vi "1_Analog_Meter_Reader(Training).vi"() -> ()   [LabVIEW 2020]
doc: "This example demonstrating the usage of Deep Learning toolkit for solving geometrical objects recognition problem based on Multilayer perceptron (MLP) and Convolutional Neural Network (CNN)."
uses:
  <vilib>/Ngene/DeepLTK/Toolkit/NN_Train/Controls/NN_LR_Policy_Cfg.ctl
  <vilib>/Ngene/DeepLTK/Toolkit/NN_Train/Controls/NN_LR_Policy_Type.ctl
  <vilib>/Ngene/DeepLTK/Toolkit/NN_Train/Controls/NN_Train_Params.ctl
  <vilib>/Ngene/DeepLTK/Toolkit/NN_Train/Controls/NN_Train_Optimizer.ctl
  <vilib>/Ngene/DeepLTK/Toolkit/NN_Train/Controls/NN_Train_Data_Sampling.ctl
  Controls/Regression_Report.ctl
  <vilib>/Ngene/DeepLTK/Toolkit/NN_Layers/Layers/FC/Controls/NN_Layer_Config(FC).ctl
  <vilib>/Ngene/DeepLTK/Toolkit/NN_Layers/Layers/BatchNorm/Controls/NN_BN_Params.ctl
  <vilib>/Ngene/DeepLTK/Toolkit/NN_Activations/Controls/NN_Activation_Type.ctl
  <vilib>/Ngene/DeepLTK/Toolkit/NN_Layers/Controls/NN_Layer_Init_Params.ctl
  <vilib>/Ngene/DeepLTK/Toolkit/NN_Layers/Controls/NN_Layer_Weight_Init_Type.ctl
  <vilib>/Ngene/DeepLTK/Toolkit/NN_Layers/Layers/Input/Controls/NN_Layer_Config(Input3D).ctl
  <vilib>/Ngene/DeepLTK/Toolkit/NN_Data/Controls/NN_Dims(C,H,W).ctl
  <vilib>/Ngene/DeepLTK/Toolkit/NN_Network/Controls/NN_Save_Before_Destroy_Options.ctl
  <vilib>/Ngene/DeepLTK/Toolkit/NN_Layers/Layers/Conv2D/Controls/NN_Layer_Config(Conv2D).ctl
  <vilib>/Ngene/DeepLTK/Toolkit/NN_Layers/Layers/Conv2D/Controls/NN_Layer_Params(Conv2D).ctl
  <vilib>/Ngene/DeepLTK/Toolkit/NN_Layers/Layers/Conv2D/Controls/NN_Conv2D_Padding_Type.ctl
  <vilib>/Ngene/DeepLTK/Toolkit/NN_Layers/Layers/DropOut3D/Controls/NN_Layer_Config(DropOut3D).ctl
  <vilib>/Ngene/DeepLTK/Toolkit/NN_Layers/Layers/Input/NN_Layer_Create(Input3D).vi
  <vilib>/Ngene/DeepLTK/Toolkit/NN_Layers/Layers/Conv2D/NN_Layer_Create(Conv2D).vi
  <vilib>/Ngene/DeepLTK/Toolkit/NN_Layers/Layers/DropOut3D/NN_Layer_Create(DropOut3D).vi
  <vilib>/Ngene/DeepLTK/Toolkit/NN_Layers/Layers/FC/NN_Layer_Create(FC).vi
  <vilib>/Ngene/DeepLTK/Toolkit/NN_Train/Loss_Functions/NN_Set_Loss(MSE).vi
  <vilib>/ptbypt/Filters.llb/FIR Filter PtByPt.vi
  <vilib>/Ngene/DeepLTK/Toolkit/NN_Network/subVIs/NN_Predict/NN_Predict(In3D_Out1D).vi
  <vilib>/Ngene/DeepLTK/Toolkit/NN_Train/Eval_Loss/NN_Eval_Test_Error_Loss/NN_Eval(In3D_Out1D).vi
  <vilib>/Ngene/DeepLTK/Toolkit/NN_Data/subVIs/Dataset_Destroy/NN_Datasets_All_Destroy(In3D_Out1D).vi
  <vilib>/Ngene/DeepLTK/Toolkit/Deep_Learning_Toolkit_by_Ngene.lvlib
panel:
  in  "NN Device":enum16{"CPU", "GPU"}(ring)=enum."GPU"
  out "Train Speed (img/s)":dbl=2338.672694098055 format="%#_3p"
  out "Train Speed (sec/batch)":dbl=0.10946379997767508 format="%#_3p"
  out "Elapsed Time":dbl=32.9020060999901 format="%<%H:%M:%S>t"
  out "Test.Dataset_Size":i32=201
  out "Train.Dataset_Size":i32=1000
  out "Loss Values":cluster{"Train_Loss":dbl, "Test_Loss":dbl}={"Train_Loss"=7.778966903686523, "Test_Loss"=0.4036712646484375} {"Test_Loss" format="%#_4g"}
  out "Session Data":T1={"Epochs"=104.19200134277344, "Tot_Iter"=407.0, "LR"=9.5367431640625e-06, "LR_iter"=408.0} {"LR" format="%#_3g"}
  out "Loss Charts":cluster{"Filtered x":sgl, "Test_Loss":sgl}(graph)={"Filtered x"=7.778967, "Test_Loss"=0.40367126}
  in  "Image Folder(Test)":path=path "D:/working/Analog_Meter/Test/Images"
  in  "Labels (Test)":path=path "D:/working/Analog_Meter/Test/Labels.csv"
  in  "Stop":bool
  out "Regression Metrics":T2={"Graphs"=[{"Best Linear Fit"=array[201 elements], "Array 3"=[2.517011, 2.0096045, 2.4545722, 2.2636914, 2.2936764, 4.560302, 5.5319304, 6.4831433, 6.3087363, 7.618647, 8.221905, 9.112002, 9.980037, 9.071789, 9.958405, 10.536366, 11.692846, 12.491657, 13.6740055, 14.302982, 14.830361, 15.396115, 15.868366, 16.362938, 16.752916, 17.515846, 18.169603, 18.99068, 19.849512, 20.732693, 21.52332, 22.002708, 22.214579, 23.227516, 24.120646, 25.386911, 25.468521, 26.268867, 27.2104, 28.526808, 28.953384, 29.351616, 29.946152, 30.505703, 31.088083, 31.950428, 32.824123, 33.49473, 34.381035, 35.134453, 35.577026, 36.282093, 36.62258, 37.27366, 37.827774, 39.678932, 40.030205, 40.623016, 41.345863, 41.777946, 42.25227, 42.78178, 43.344627, 44.43666, 45.447147, 46.357304, 47.180454, 47.77743, 48.22017, 48.731907, 49.320972, 50.022675, 50.477943, 51.13582, 51.981068, 52.795086, 53.414444, 54.063515, 54.653965, 56.161224, 56.6563, 57.51746, 58.014706, 58.689663, 59.56889, 60.116806, 60.655125, 61.062958, 61.754738, 62.627365, 63.322636, 63.751377, 64.42173, 65.163635, 65.93629, 67.140495, 67.96894, 68.54193, 69.32477, 69.879906, 70.43094, 71.16161, 71.60928, 72.36131, 72.99475, 73.651764, 74.624405, 75.3703, 76.09268, 76.79159, 77.39567, 78.15343, 78.86843, 79.65233, 80.15797, 80.81467, 81.317024, 82.1362, 82.814064, 83.34939, 84.02449, 84.577354, 86.16109, 86.68068, 87.33571, 88.01903, 88.70086, 89.229324, 89.99918, 90.731285, 91.37161, 92.006744, 92.70506, 93.25279, 94.06685, 94.801796, 95.546906, 96.167404, 97.10623, 97.73104, 98.33137, 98.990654, 99.54073, 100.25781, 100.895294, 101.526665, 102.33004, 102.97929, 103.77419, 104.16804, 104.88838, 106.019455, 106.816345, 107.406876, 108.19176, 109.02587, 109.658844, 110.24592, 110.704124, 111.26262, 111.76719, 112.43235, 113.87547, 114.76889, 115.557724, 115.86315, 116.95176, 117.768394, 118.702324, 118.6948, 119.12609, 119.788155, 120.696465, 121.51759, 122.282455, 122.96412, 123.52434, 124.11557, 124.71953, 125.29246, 125.93008, 126.66733, 127.38417, 128.6919, 129.43976, 130.39424, 131.04564, 131.64711, 131.56487, 132.2587, 133.19635, 133.81221, 134.28249, 134.72006, 135.67499, 136.66454, 138.42493, 138.63422, 138.48953, 138.73322, 137.90044]}, {"Best Linear Fit"=array[201 elements], "Array 3"=[2.517011, 2.0096045, 2.4545722, 2.2636914, 2.2936764, 4.560302, 5.5319304, 6.4831433, 6.3087363, 7.618647, 8.221905, 9.112002, 9.980037, 9.071789, 9.958405, 10.536366, 11.692846, 12.491657, 13.6740055, 14.302982, 14.830361, 15.396115, 15.868366, 16.362938, 16.752916, 17.515846, 18.169603, 18.99068, 19.849512, 20.732693, 21.52332, 22.002708, 22.214579, 23.227516, 24.120646, 25.386911, 25.468521, 26.268867, 27.2104, 28.526808, 28.953384, 29.351616, 29.946152, 30.505703, 31.088083, 31.950428, 32.824123, 33.49473, 34.381035, 35.134453, 35.577026, 36.282093, 36.62258, 37.27366, 37.827774, 39.678932, 40.030205, 40.623016, 41.345863, 41.777946, 42.25227, 42.78178, 43.344627, 44.43666, 45.447147, 46.357304, 47.180454, 47.77743, 48.22017, 48.731907, 49.320972, 50.022675, 50.477943, 51.13582, 51.981068, 52.795086, 53.414444, 54.063515, 54.653965, 56.161224, 56.6563, 57.51746, 58.014706, 58.689663, 59.56889, 60.116806, 60.655125, 61.062958, 61.754738, 62.627365, 63.322636, 63.751377, 64.42173, 65.163635, 65.93629, 67.140495, 67.96894, 68.54193, 69.32477, 69.879906, 70.43094, 71.16161, 71.60928, 72.36131, 72.99475, 73.651764, 74.624405, 75.3703, 76.09268, 76.79159, 77.39567, 78.15343, 78.86843, 79.65233, 80.15797, 80.81467, 81.317024, 82.1362, 82.814064, 83.34939, 84.02449, 84.577354, 86.16109, 86.68068, 87.33571, 88.01903, 88.70086, 89.229324, 89.99918, 90.731285, 91.37161, 92.006744, 92.70506, 93.25279, 94.06685, 94.801796, 95.546906, 96.167404, 97.10623, 97.73104, 98.33137, 98.990654, 99.54073, 100.25781, 100.895294, 101.526665, 102.33004, 102.97929, 103.77419, 104.16804, 104.88838, 106.019455, 106.816345, 107.406876, 108.19176, 109.02587, 109.658844, 110.24592, 110.704124, 111.26262, 111.76719, 112.43235, 113.87547, 114.76889, 115.557724, 115.86315, 116.95176, 117.768394, 118.702324, 118.6948, 119.12609, 119.788155, 120.696465, 121.51759, 122.282455, 122.96412, 123.52434, 124.11557, 124.71953, 125.29246, 125.93008, 126.66733, 127.38417, 128.6919, 129.43976, 130.39424, 131.04564, 131.64711, 131.56487, 132.2587, 133.19635, 133.81221, 134.28249, 134.72006, 135.67499, 136.66454, 138.42493, 138.63422, 138.48953, 138.73322, 137.90044]}, {"Best Linear Fit"=[0.0, 140.0], "Array 3"=[0.0, 140.0]}], "y=k*x+b"="y = 0.996*x + 0.683", "R"=0.9999493, "R^2"=0.99989855, "MAE"=0.46021813, "MSE"=0.3585698} {"R" format="%#_7g"}
  in  "Evaluate Model":bool
  in  "LR Update Policy":T3={"Policy_Type"=enum."Step", "LR0"=10.0, "k"=5.0, "WarmUp_Policy"=enum."Ramp", "WarmUp_Iter"=50, "WarmUp_Ratio"=50.0} {"WarmUp_Ratio" min=1; "WarmUp_Iter" min=1; "LR0" format="%.7f"}
  in  "Train_Params":T5={"Optimizer"=enum."Adam", "Beta_1"=0.9, "Beta_2"=0.999, "Weight Decay(L1)"=7e-09, "Weight Decay(L2)"=7e-09, "Data_Sampling"=enum."Random"}
  in  "Image Folder(Train)":path=path "D:/working/Analog_Meter/Train/Images"
  in  "Labels (Train)":path=path "D:/working/Analog_Meter/Train/Labels.csv"
  in  "Input Height":i32=256
  in  "Input Width":i32=256
  out "Test_Loss":sgl=0.35856977
  # "Overview: This example project demonstrates the usage of Deep Learning Toolkit for solving Image Regression, specifically creating analog meter reader. \nRequirements: DeepLTK (Deep Learning Toolkit for LabVIEW) - https://www.ngene.co/deep-learning-toolkit-for-labview\nInstructions:\n1.Provide Generated dataset paths to the VI.\n2.Run the VI with current configuration of the training parameters and Learning Rate update policy.\n3.Observe the Loss Charts, how the train and test losses are decreasing.\n4. Stop the VI, if the train loss isn't decreasing anymore (about 100 epochs)."
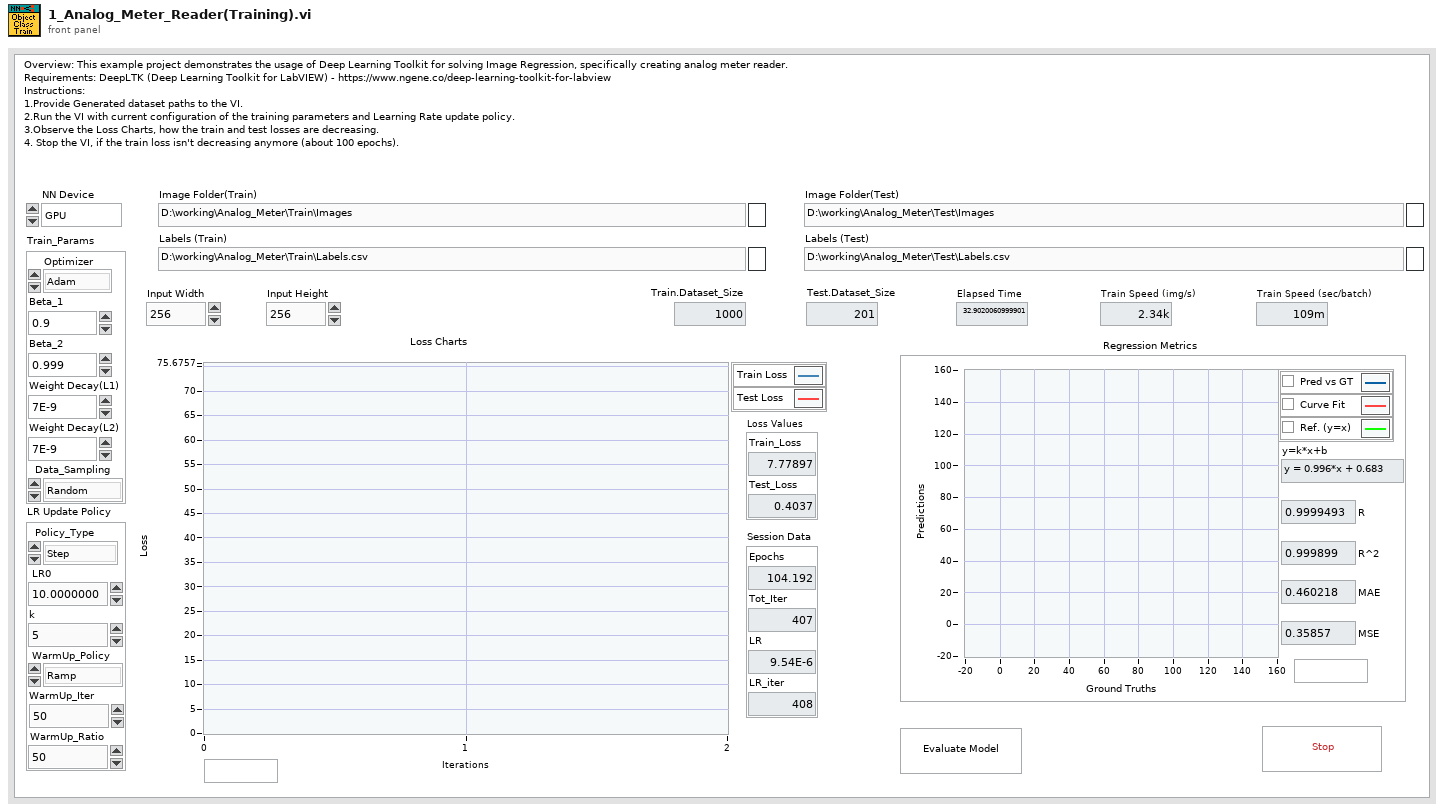
[diagram p1: front panel]
types:
  T1 = cluster{"Epochs":dbl, "Tot_Iter":dbl, "LR":dbl, "LR_iter":dbl}
  T2 = typedef "Regression_Report.ctl" = cluster{"Graphs":cluster{"Best Linear Fit":dbl[], "Array 3":sgl[]}[], "y=k*x+b":string, "R":sgl, "R^2":sgl, "MAE":sgl, "MSE":sgl}
  T3 = typedef "Deep_Learning_Toolkit_by_Ngene.lvlib/NN_LR_Policy_Cfg.ctl" = cluster{"Policy_Type":T4, "LR0":dbl, "k":sgl, "WarmUp_Policy":enum16{"Step", "Ramp"}, "WarmUp_Iter":i32, "WarmUp_Ratio":sgl}
  T4 = typedef "Deep_Learning_Toolkit_by_Ngene.lvlib/NN_LR_Policy_Type.ctl" = enum16{"Manual", "Step", "Exp", "1/t"}
  T5 = typedef "Deep_Learning_Toolkit_by_Ngene.lvlib/NN_Train_Params.ctl" = cluster{"Optimizer":T6, "Beta_1":sgl, "Beta_2":sgl, "Weight Decay(L1)":sgl, "Weight Decay(L2)":sgl, "Data_Sampling":T7}
  T6 = typedef "Deep_Learning_Toolkit_by_Ngene.lvlib/NN_Train_Optimizer.ctl" = enum16{"SGD", "Adam", "Adagrad", "Adadelta", "RMSProp", "Nesterov"}
  T7 = typedef "Deep_Learning_Toolkit_by_Ngene.lvlib/NN_Train_Data_Sampling.ctl" = enum16{"Random", "Sequential"}
  T8 = typedef "Deep_Learning_Toolkit_by_Ngene.lvlib/NN_Layer_Config(Conv2D).ctl" = cluster{"Name":string, "Conv_Params":T9, "BN?":bool, "BN_Params":T11, "Activation":T12, "Has Bias?":bool, "Init_Params":T13, "Custom_Params":string}
  T9 = typedef "Deep_Learning_Toolkit_by_Ngene.lvlib/NN_Layer_Params(Conv2D).ctl" = cluster{"Filters":i32, "Kernel_Size":i32, "Stride":i32, "Pad_Type":T10, "Pad_Size":i32}
  T10 = typedef "Deep_Learning_Toolkit_by_Ngene.lvlib/NN_Conv2D_Padding_Type.ctl" = enum16{"Pad_Size", "Valid", "Same"}
  T11 = typedef "Deep_Learning_Toolkit_by_Ngene.lvlib/NN_BN_Params.ctl" = cluster{"epsilon":sgl, "momentum":sgl}
  T12 = typedef "Deep_Learning_Toolkit_by_Ngene.lvlib/NN_Activation_Type.ctl" = enum16{"Sigmoid", "ReLU", "LReLU", "ReLU6", "tanh", "Swish", "Mish", "None"}
  T13 = typedef "Deep_Learning_Toolkit_by_Ngene.lvlib/NN_Layer_Init_Params.ctl" = cluster{"Init_Type":T14, "Value":sgl}
  T14 = typedef "Deep_Learning_Toolkit_by_Ngene.lvlib/NN_Layer_Weight_Init_Type.ctl" = enum16{"Const", "Uniform", "Gaussian", "Xavier"}
  T15 = typedef "Deep_Learning_Toolkit_by_Ngene.lvlib/NN_Layer_Config(DropOut3D).ctl" = cluster{"Name":string, "Probability":sgl}
  T16 = typedef "Deep_Learning_Toolkit_by_Ngene.lvlib/NN_Layer_Config(FC).ctl" = cluster{"Name":string, "Size":i32, "BN":bool, "BN_Params":T11, "Activation":T12, "Has Bias?":bool, "Init_Params":T13, "Custom_Params":string}
  T17 = typedef "Deep_Learning_Toolkit_by_Ngene.lvlib/NN_Save_Before_Destroy_Options.ctl" = cluster{"CFG?":bool, "Weights?":bool, "Render?":bool}
  T18 = typedef "Deep_Learning_Toolkit_by_Ngene.lvlib/NN_Layer_Config(Input3D).ctl" = cluster{"Name":string, "Dims":T19}
  T19 = typedef "Deep_Learning_Toolkit_by_Ngene.lvlib/NN_Dims(C,H,W).ctl" = cluster{"C":i32, "H":i32, "W":i32}
  T20 = typedef "Deep_Learning_Toolkit_by_Ngene.lvlib/NN_DataSets_All(In3D_Out1D).ctl" = cluster{"Train":T21, "Validation":T21, "Test":T21}
  T21 = typedef "Deep_Learning_Toolkit_by_Ngene.lvlib/NN_DataSet(In3D_Out1D).ctl" = cluster{"Inputs Ref.":T22, "Outputs Ref.":T23, "Dataset_Size":i32, "Dims_In":T19, "Dims_Out":i32, "Labels":string[], "File Paths":path[]}
  T22 = typedef "Deep_Learning_Toolkit_by_Ngene.lvlib/NN_Data_ref(4D_SGL).ctl" = refnum<data-value>
  T23 = typedef "Deep_Learning_Toolkit_by_Ngene.lvlib/NN_Data_ref(2D_SGL).ctl" = refnum<data-value>
  T24 = typedef "Deep_Learning_Toolkit_by_Ngene.lvlib/NN.ctl" = cluster{"Name":string, "No of Layers":i32, "mBatch":i32, "Layers":T25[], "Dimty":T26, "Dims_In":T19, "Dims_Out":T19, "Working_Dir":path, "Train?":bool, "Train_Params":T5, "LR_Update_Policy":T3, "Session Data":T27, "Ground_truth":T28, "NNg_hdls":T29, "NN_Device":T30, "GPU Id":i32, "Labels":string[], "Receptive Field":T31[], "Loss_Type":T32, "Loss_Cfg_Prms":variant, "NNG_WS":T33}
  T25 = typedef "Deep_Learning_Toolkit_by_Ngene.lvlib/NN_Layer_ref.ctl" = refnum<data-value>
  T26 = typedef "Deep_Learning_Toolkit_by_Ngene.lvlib/NN_In_Out_Dim-ty.ctl" = enum8{"In1D_Out1D", "In3D_Out1D", "In3D_Out3D", "In3D_OutBBox"}
  T27 = typedef "Deep_Learning_Toolkit_by_Ngene.lvlib/NN_Train_Session_Data.ctl" = cluster{"Epochs":sgl, "Tot_Iter":i32, "LR":sgl, "LR_iter":i32}
  T28 = typedef "Deep_Learning_Toolkit_by_Ngene.lvlib/NN_Ground_truth.ctl" = cluster{"Y":variant}
  T29 = typedef "Deep_Learning_Toolkit_by_Ngene.lvlib/nng_cuda_handles.ctl" = cluster{"cudnn":u64, "cublas":u64, "stream":u64, "curand":u64}
  T30 = typedef "Deep_Learning_Toolkit_by_Ngene.lvlib/NN_Device.ctl" = enum16{"CPU", "GPU"}
  T31 = typedef "Deep_Learning_Toolkit_by_Ngene.lvlib/NN_Dims(V,H).ctl" = cluster{"V":i32, "H":i32}
  T32 = typedef "Deep_Learning_Toolkit_by_Ngene.lvlib/NN_Loss_Type.ctl" = enum16{"None", "MSE", "CrossEntropy", "YOLO_v2", "YOLO_v4"}
  T33 = typedef "Deep_Learning_Toolkit_by_Ngene.lvlib/NNG_WS.ctl" = cluster{"NNG_WS_Mem":T34, "Max_WS_Size":i64}
  T34 = typedef "Deep_Learning_Toolkit_by_Ngene.lvlib/NNg_WS_Mem_DVR.ctl" = refnum<data-value>
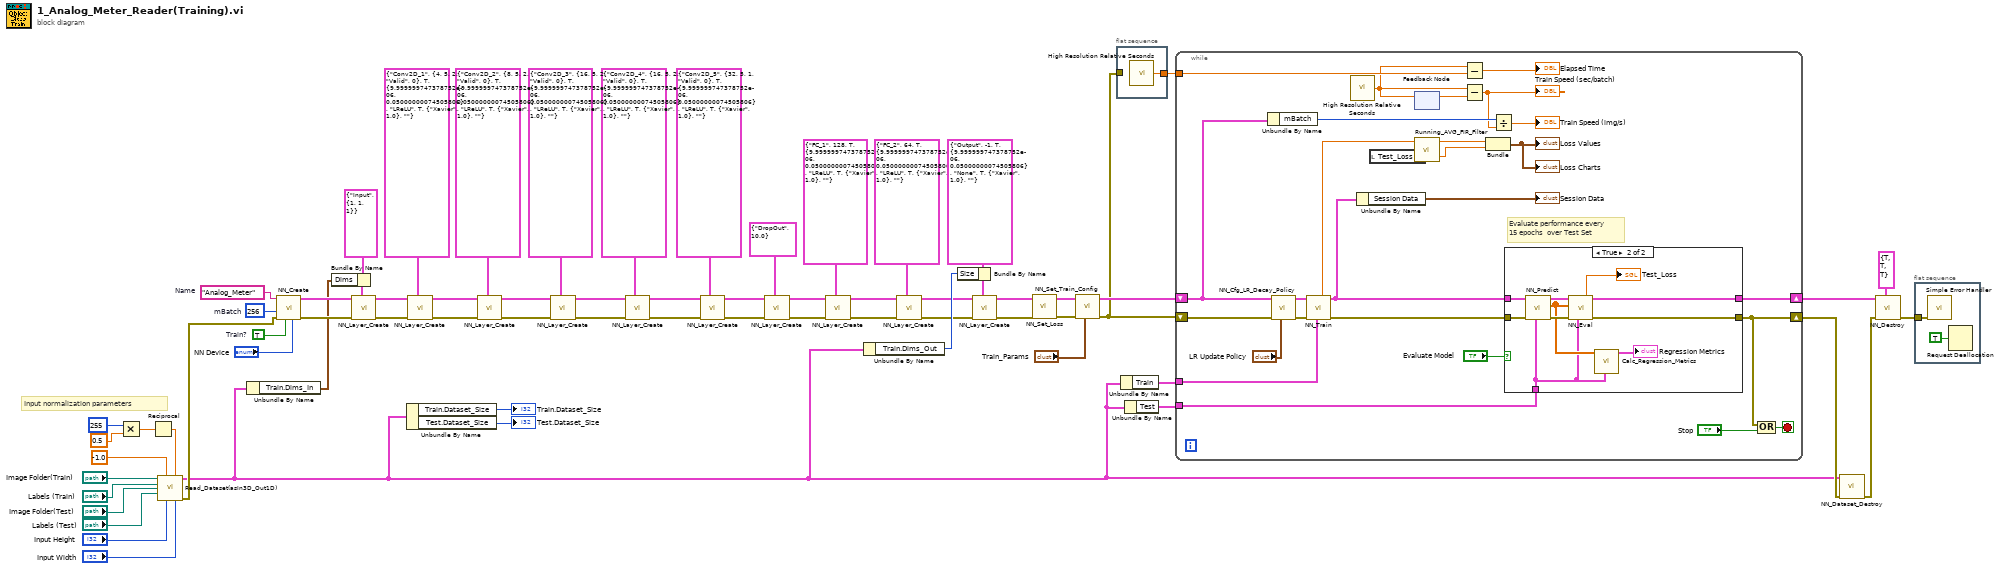
[diagram p0: block diagram]
diagram:
  w50 = TRUE  # Train?
  w62 = 256  # mBatch
  w67 = "Analog_Meter"  # Name
  # "Input normalization parameters"
  n1 = Multiply(x=u16 255 ("Shift"), y=sgl 0.5 ("Scale")) -> (x*y=w23:sgl)
  n2 = Reciprocal(x=w23) -> (1/x=w22:sgl)
  n3 = call "Read_Dataset(asIn3D_Out1D).vi"("Image Folder Path(Train)"="Image Folder(Train)", "Norm. Shift"=sgl -1.0 ("Scale"), "Norm. Scale"=w22, "Label File Path(Train)"="Labels (Train)", "Image Folder Path(Test)"="Image Folder(Test)", "Label File Path(Test)"="Labels (Test)", "Img Heigth"="Input Height", "Img Width"="Input Width") -> ("Datasets"=w6:T20, "error out"=w68:errorcluster)  [unwired: 6 in]
  n4 = Unbundle By Name(w6) -> ("Train.Dims_In"=w45:T19)
  n5 = call <vilib>:"NN_Create.vi"("NN_Device"="NN Device", "Train? (false)"=w50, "error in (no error)"=w68, "mBatch (1)"=w62, "Name"=w67) -> ("error out"=w65:errorcluster, "NN out"=w66:T24)  [unwired: 5 in]
  n6 = Bundle By Name(cluster=T18 {"Name"="Input", "Dims"={"C"=1, "H"=1, "W"=1}} ("Cluster"), "Dims"=w45) -> (w53:T18)
  n7 = call-poly <vilib>:"NN_Layer_Create.vi"("Input3D_Cfg"=w53, "error in (no error)"=w65, "NN In"=w66) -> ("error out"=w59:errorcluster, "NN out"=w60:T24)  [unwired: 6 in, 1 out]
  n8 = Unbundle By Name(w6) -> ("Train.Dataset_Size"=→"Train.Dataset_Size":i32, "Test.Dataset_Size"=→"Test.Dataset_Size":i32)
  n9 = call-poly <vilib>:"NN_Layer_Create.vi"("Conv2D_Cfg"=T8 {"Name"="Conv2D_1", "Conv_Params"={"Filters"=4, "Kernel_Size"=5, "Stride"=2, "Pad_Type"=enum."Valid", "Pad_Size"=0}, "BN?"=TRUE, "BN_Params"={"epsilon"=1e-05, "momentum"=0.05}, "Activation"=enum."LReLU", "Has Bias?"=TRUE, "Init_Params"={"Init_Type"=enum."Xavier", "Value"=1.0}, "Custom_Params"=""}, "error in (no error)"=w59, "NN in"=w60) -> ("error out"=w19:errorcluster, "NN out"=w18:T24)  [unwired: 6 in, 1 out]
  n10 = call-poly <vilib>:"NN_Layer_Create.vi"("Conv2D_Cfg"=T8 {"Name"="Conv2D_2", "Conv_Params"={"Filters"=8, "Kernel_Size"=5, "Stride"=2, "Pad_Type"=enum."Valid", "Pad_Size"=0}, "BN?"=TRUE, "BN_Params"={"epsilon"=1e-05, "momentum"=0.05}, "Activation"=enum."LReLU", "Has Bias?"=TRUE, "Init_Params"={"Init_Type"=enum."Xavier", "Value"=1.0}, "Custom_Params"=""}, "error in (no error)"=w19, "NN in"=w18) -> ("error out"=w42:errorcluster, "NN out"=w43:T24)  [unwired: 6 in, 1 out]
  n11 = call-poly <vilib>:"NN_Layer_Create.vi"("Conv2D_Cfg"=T8 {"Name"="Conv2D_3", "Conv_Params"={"Filters"=16, "Kernel_Size"=5, "Stride"=2, "Pad_Type"=enum."Valid", "Pad_Size"=0}, "BN?"=TRUE, "BN_Params"={"epsilon"=1e-05, "momentum"=0.05}, "Activation"=enum."LReLU", "Has Bias?"=TRUE, "Init_Params"={"Init_Type"=enum."Xavier", "Value"=1.0}, "Custom_Params"=""}, "error in (no error)"=w42, "NN in"=w43) -> ("error out"=w10:errorcluster, "NN out"=w11:T24)  [unwired: 6 in, 1 out]
  n12 = call-poly <vilib>:"NN_Layer_Create.vi"("Conv2D_Cfg"=T8 {"Name"="Conv2D_4", "Conv_Params"={"Filters"=16, "Kernel_Size"=5, "Stride"=2, "Pad_Type"=enum."Valid", "Pad_Size"=0}, "BN?"=TRUE, "BN_Params"={"epsilon"=1e-05, "momentum"=0.05}, "Activation"=enum."LReLU", "Has Bias?"=TRUE, "Init_Params"={"Init_Type"=enum."Xavier", "Value"=1.0}, "Custom_Params"=""}, "error in (no error)"=w10, "NN in"=w11) -> ("error out"=w3:errorcluster, "NN out"=w4:T24)  [unwired: 6 in, 1 out]
  n13 = call-poly <vilib>:"NN_Layer_Create.vi"("Conv2D_Cfg"=T8 {"Name"="Conv2D_5", "Conv_Params"={"Filters"=32, "Kernel_Size"=5, "Stride"=1, "Pad_Type"=enum."Valid", "Pad_Size"=0}, "BN?"=TRUE, "BN_Params"={"epsilon"=1e-05, "momentum"=0.05}, "Activation"=enum."LReLU", "Has Bias?"=TRUE, "Init_Params"={"Init_Type"=enum."Xavier", "Value"=1.0}, "Custom_Params"=""}, "error in (no error)"=w3, "NN in"=w4) -> ("error out"=w1:errorcluster, "NN out"=w2:T24)  [unwired: 6 in, 1 out]
  n14 = call-poly <vilib>:"NN_Layer_Create.vi"("DropOut3D_Cfg"=T15 {"Name"="DropOut", "Probability"=10.0}, "error in (no error)"=w1, "NN in"=w2) -> ("error out"=w8:errorcluster, "NN out"=w9:T24)  [unwired: 6 in, 1 out]
  n15 = call-poly <vilib>:"NN_Layer_Create.vi"("FC_Cfg"=T16 {"Name"="FC_1", "Size"=128, "BN"=TRUE, "BN_Params"={"epsilon"=1e-05, "momentum"=0.05}, "Activation"=enum."LReLU", "Has Bias?"=TRUE, "Init_Params"={"Init_Type"=enum."Xavier", "Value"=1.0}, "Custom_Params"=""} ("Layer_Config_Params"), "error in (no error)"=w8, "NN in"=w9) -> ("error out"=w20:errorcluster, "NN out"=w21:T24)  [unwired: 6 in, 1 out]
  n16 = Unbundle By Name(w6) -> ("Train.Dims_Out"=w44:i32)
  n17 = call-poly <vilib>:"NN_Layer_Create.vi"("FC_Cfg"=T16 {"Name"="FC_2", "Size"=64, "BN"=TRUE, "BN_Params"={"epsilon"=1e-05, "momentum"=0.05}, "Activation"=enum."LReLU", "Has Bias?"=TRUE, "Init_Params"={"Init_Type"=enum."Xavier", "Value"=1.0}, "Custom_Params"=""} ("Layer_Config_Params"), "error in (no error)"=w20, "NN in"=w21) -> ("error out"=w25:errorcluster, "NN out"=w26:T24)  [unwired: 6 in, 1 out]
  n18 = Bundle By Name(cluster=T16 {"Name"="Output", "Size"=-1, "BN"=TRUE, "BN_Params"={"epsilon"=1e-05, "momentum"=0.05}, "Activation"=enum."None", "Has Bias?"=TRUE, "Init_Params"={"Init_Type"=enum."Xavier", "Value"=1.0}, "Custom_Params"=""} ("Layer_Config_Params"), "Size"=w44) -> (w54:T16)
  n19 = call-poly <vilib>:"NN_Layer_Create.vi"("FC_Cfg"=w54, "error in (no error)"=w25, "NN in"=w26) -> ("error out"=w57:errorcluster, "NN out"=w58:T24)  [unwired: 6 in, 1 out]
  n20 = call-poly <vilib>:"NN_Set_Loss.vi"("error in (no error)"=w57, "NN in"=w58) -> ("error out"=w37:errorcluster, "NN out"=w38:T24)  [unwired: 8 in]
  n21 = call <vilib>:"NN_Set_Train_Config.vi"("NN_Train_Params"="Train_Params", "error in (no error)"=w37, "NN in"=w38) -> ("error out"=w51:errorcluster, "NN out"=w52:T24)  [unwired: 7 in]
  n22 = flat-sequence {
    tunnel: [w69] -> w64
    tunnel: w51 -> [_]
    frame #0 {
      n23 = call <vilib>:"High Resolution Relative Seconds.vi"() -> ("relative seconds"=w69:dbl)
    }
  }
  n24 = Unbundle By Name(w6) -> ("Train"=w48:T21)
  n25 = Unbundle By Name(w6) -> ("Test"=w61:T21)
  n26 = while {
    shift-right: [w71] -> w36
    shift-left: w51 -> [w80]
    shift-right: [w72] -> w35
    shift-left: w52 -> [w81]
    tunnel: w64 -> [w87]
    tunnel: w48 -> [w78]
    tunnel: w61 -> [w83]
    stop <- w93 stop-if-true
    # "Evaluate performance every\n15 epochs  over Test Set"
    n27 = Unbundle By Name(w81) -> ("mBatch"=w85:i32)
    n28 = call <vilib>:"NN_Cfg_LR_Decay_Policy.vi"("LR_Decay_Params"="LR Update Policy", "error in (no error)"=w80, "NN in"=w81) -> ("error out"=w88:errorcluster, "NN out"=w94:T24)  [unwired: 7 in]
    n29 = call <vilib>:"NN_Train.vi"("Train Dataset"=w78, "error in (no error)"=w88, "NN in"=w94) -> ("error out"=w84:errorcluster, "NN out"=w79:T24, "Loss"=w89:sgl)  [unwired: 4 in, 2 out]
    n30 = call <vilib>:"High Resolution Relative Seconds.vi"() -> ("relative seconds"=w86:dbl)
    n31 = Unbundle By Name(w79) -> ("Session Data"=→"Session Data":T27)
    n32 = local read "Test_Loss"() -> (w92:sgl)
    n33 = feedback #1() -> (w95:dbl)  [unwired: 1 in]
    n34 = feedback-in #1(w86) -> ()
    n35 = call <vilib>:"Running_AVG_FIR_Filter.vi"("Numeric"=w89) -> ("Filtered x"=w90:sgl)  [unwired: 10 in]
    n36 = Subtract(x=w86, y=w87) -> (x-y=→"Elapsed Time":dbl)
    n37 = Subtract(x=w86, y=w95) -> (x-y=w75:dbl)
    "Train Speed (sec/batch)" <- w75
    n38 = Bundle("Filtered x"=w90, "Test_Loss"=w92) -> (→"Loss Values" →"Loss Charts":cluster{"Filtered x":sgl, "Test_Loss":sgl})  [unwired: 1 in]
    n39 = Divide(x=w85, y=w75) -> (x/y=→"Train Speed (img/s)":dbl)
    n40 = case shown="True" "Evaluate Model" {
      tunnel: w79 -> [w96 w107]
      tunnel: w84 -> [w97 w102]
      tunnel: [w97 w104] -> w71
      tunnel: w83 -> [_ w98]
      tunnel: [w96 w105] -> w72
      frame False {
      }
      frame True {
        n41 = call-poly <vilib>:"NN_Predict.vi"("Dataset"=w98, "error in (no error)"=w102, "NN in"=w107) -> ("error out"=w101:errorcluster, "Predictions"=w100:sgl[][], "NN out"=w103:T24)  [unwired: 6 in]
        n42 = call-poly <vilib>:"NN_Eval.vi"("NN in"=w103, "Predictions"=w100, "error in (no error)"=w101, "Dataset"=w98) -> ("Loss"=→"Test_Loss":sgl, "NN out"=w105:T24, "error out"=w104:errorcluster)  [unwired: 7 in, 2 out]
        n43 = call "Calc_Regression_Metrics.vi"("Dataset"=w98, "Predictions"=w100) -> ("Metrics"=→"Regression Metrics":T2)  [unwired: 9 in]
      }
    }
    n44 = Compound Arithmetic op=OR(w71, "Stop") -> (w93:bool)
  }
  n45 = call-poly <vilib>:"NN_Dataset_Destroy.vi"("error in (no error)"=w36, "Datasets_All(In3D_Out1D)"=w6) -> ("error out"=w34:errorcluster)  [unwired: 9 in]
  n46 = call <vilib>:"NN_Destroy.vi"("Save (T, T, T)"=T17 {"CFG?"=TRUE, "Weights?"=TRUE, "Render?"=TRUE} ("Save_Config"), "error in (no error)"=w34, "NN in"=w35) -> ("error out"=w46:errorcluster)  [unwired: 7 in, 1 out]
  n47 = flat-sequence {
    tunnel: w46 -> [w109]
    frame #0 {
      n48 = call <vilib>:"Simple Error Handler.vi"("error in (no error)"=w109) -> ()  [unwired: 4 in, 5 out]
      n49 = Request Deallocation(TRUE ("flag")) -> ()
    }
  }
